vi "12 - Design Pattern - Reusable Event Handlers (as a Brat VI).vi"() -> ()   [LabVIEW 2012]
panel:
  out "Relayed event":i32
  in  "Generate Event to Delegate":bool
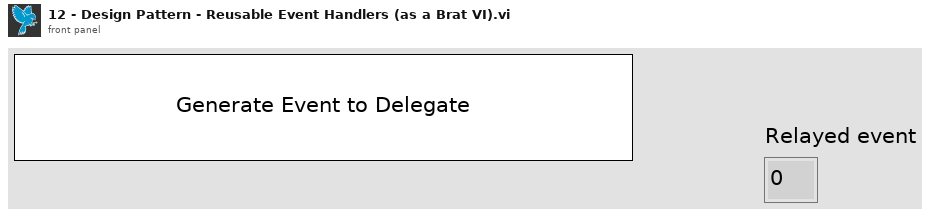
[diagram p1: front panel]
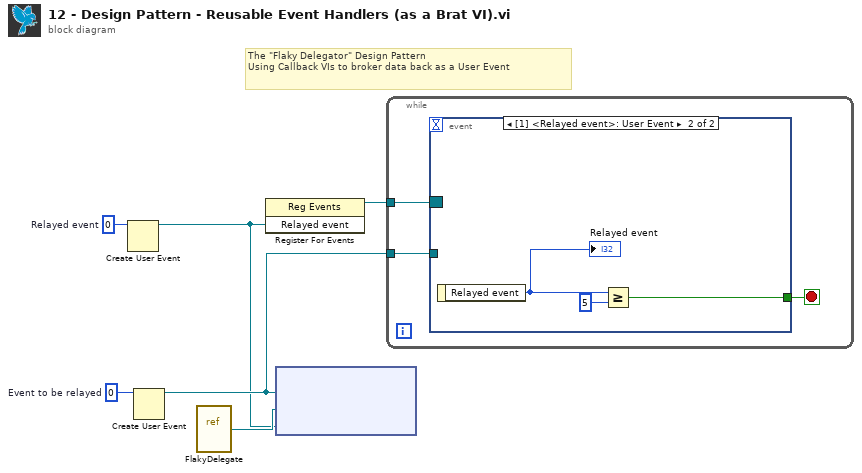
[diagram p0: block diagram]
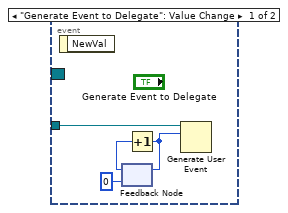
[diagram p2: hidden frame]
diagram:
  w5 = 0  # Relayed event
  w6 = 0  # Event to be relayed
  # "The \"Flaky Delegator\" Design Pattern\nUsing Callback VIs to broker data back as a User Event"
  n1 = Create User Event(user event datatype=w5) -> (user event=w2:refnum<user-event>)  [unwired: 1 in, 1 out]
  n2 = Create User Event(user event datatype=w6) -> (user event=w4:refnum<user-event>)  [unwired: 1 in, 1 out]
  n3 = vi-ref "FlakyDelegate.vi"() -> ("vi reference"=w3:refnum<vi>)
  n4 = register-events(w2) -> (reference out=w1:refnum<event-registration>)  [unwired: 2 in, 1 out]
  n5 = node(w4, w3, w2) -> ()  [unwired: 2 in, 2 out]
  n6 = while {
    tunnel: w4 -> [w9]
    tunnel: w1 -> [w7]
    stop <- w8 stop-if-true
    n7 = event shown="[1] <Relayed event>: User Event" {
      selector: w7 -> [_ _]
      dyn-events: _ -> [_ _]
      timeout: _ -> [_ _]
      tunnel: w9 -> [w13 _]
      tunnel: [_ w14] -> w8
      event "Generate Event to Delegate": Value Change {
        n8 = event-data() -> ()  [unwired: 1 in, 1 out]
        n9 = feedback #1(0) -> (w12:i32)
        n10 = Increment(x=w12) -> (x+1=w10:i32)
        n11 = feedback-in #1(w10) -> ()
        n12 = Generate User Event(user event=w13, event data cluster=w10) -> ()  [unwired: 1 in, 2 out]
      }
      event User Event {
        n13 = event-data() -> ("Relayed event"=w16:i32)  [unwired: 1 in]
        "Relayed event" <- w16
        n14 = Greater Or Equal?(x=w16, y=5) -> (x >= y?=w14:bool)
      }
    }
  }
